vi "TallGuants_Main.vi"() -> ()   [LabVIEW 2017]
doc: "Use this template to build a simple state machine design pattern. Each state executes code and determines which state to transition to."
uses:
  controls/State.ctl
  controls/Data.ctl
  <vilib>/Utility/file.llb/Write Delimited Spreadsheet (string).vi
panel:
  in  "Sortir":bool caption="SALIR"
  out "Password":string
  out "EstatMaquina1":T1
  out "ParoEmergencia":bool caption="Paro de\nEmergencia"
  out "Retenida":bool
  out "Ensayo activo":bool caption="Prueba en marcha"
  out "Liberada":bool
  out "FCI":bool
  out "FCS":bool
  out "ADFet":bool
  out "CalibratgeDefor":dbl
  out "NProves":u8 caption="Longitud de corte"
  out "ValorSenseTara":dbl
  out "EntradesD":bool[](array[boolean])
  out "SortidesD":bool[](array[boolean])
  out "UI":bool[](array[boolean])
  in  "Vel.Maxima":sgl caption="Longitud de corte" format="%.1f"
  in  "Velocitat":sgl caption="Longitud de corte" format="%.1f"
  out "DadesAD":cluster{"Dades":sgl, "data":bool[]}
  in  "data":bool[](array[boolean])
  in  "Dades":sgl caption="Longitud de corte" format="%.1f"
  out "DigitalIn":refnum<vi>[](array[refnum])
  out "Tall":bool caption="Liberada"
  out "LongitudSenseTara":sgl caption="Longitud de corte" format="%.1f"
  out "Exit":bool
  out "FactorsUnitatsPendents_D":dbl[](array[numeric])
  out "ConversioUnitatsD":dbl[](array[numeric])=[1.0, 9.8756, 1000.0, 0.98]
  out "Tara":sgl caption="Longitud de corte" format="%.1f"
  in  "Table Control":string[][](table)
  in  "EnsayoNuevo":bool caption="Ensayo nuevo"
  in  "Calibracion":bool caption="Configuración"
  in  "Informe":bool
  in  "Fuerza de corte (N)":u16(ring) items=["1", "22", "33", "44", "5", "6", "7", "8", "9", "10", "11", "12", "13", "14", "15", "16", "17", "18", "19", "20", "21", "22", "23", "24", "25", "26", "27", "28", "29", "30"]
  in  "Down":bool
  in  "UP":bool caption="Up"
  in  "Cuchilla":bool
  in  "UnidadesD":u16(ring) caption="Unidades" items=["mm", "inch"]
  out "Longitud":sgl caption="Longitud de corte" format="%.2f"
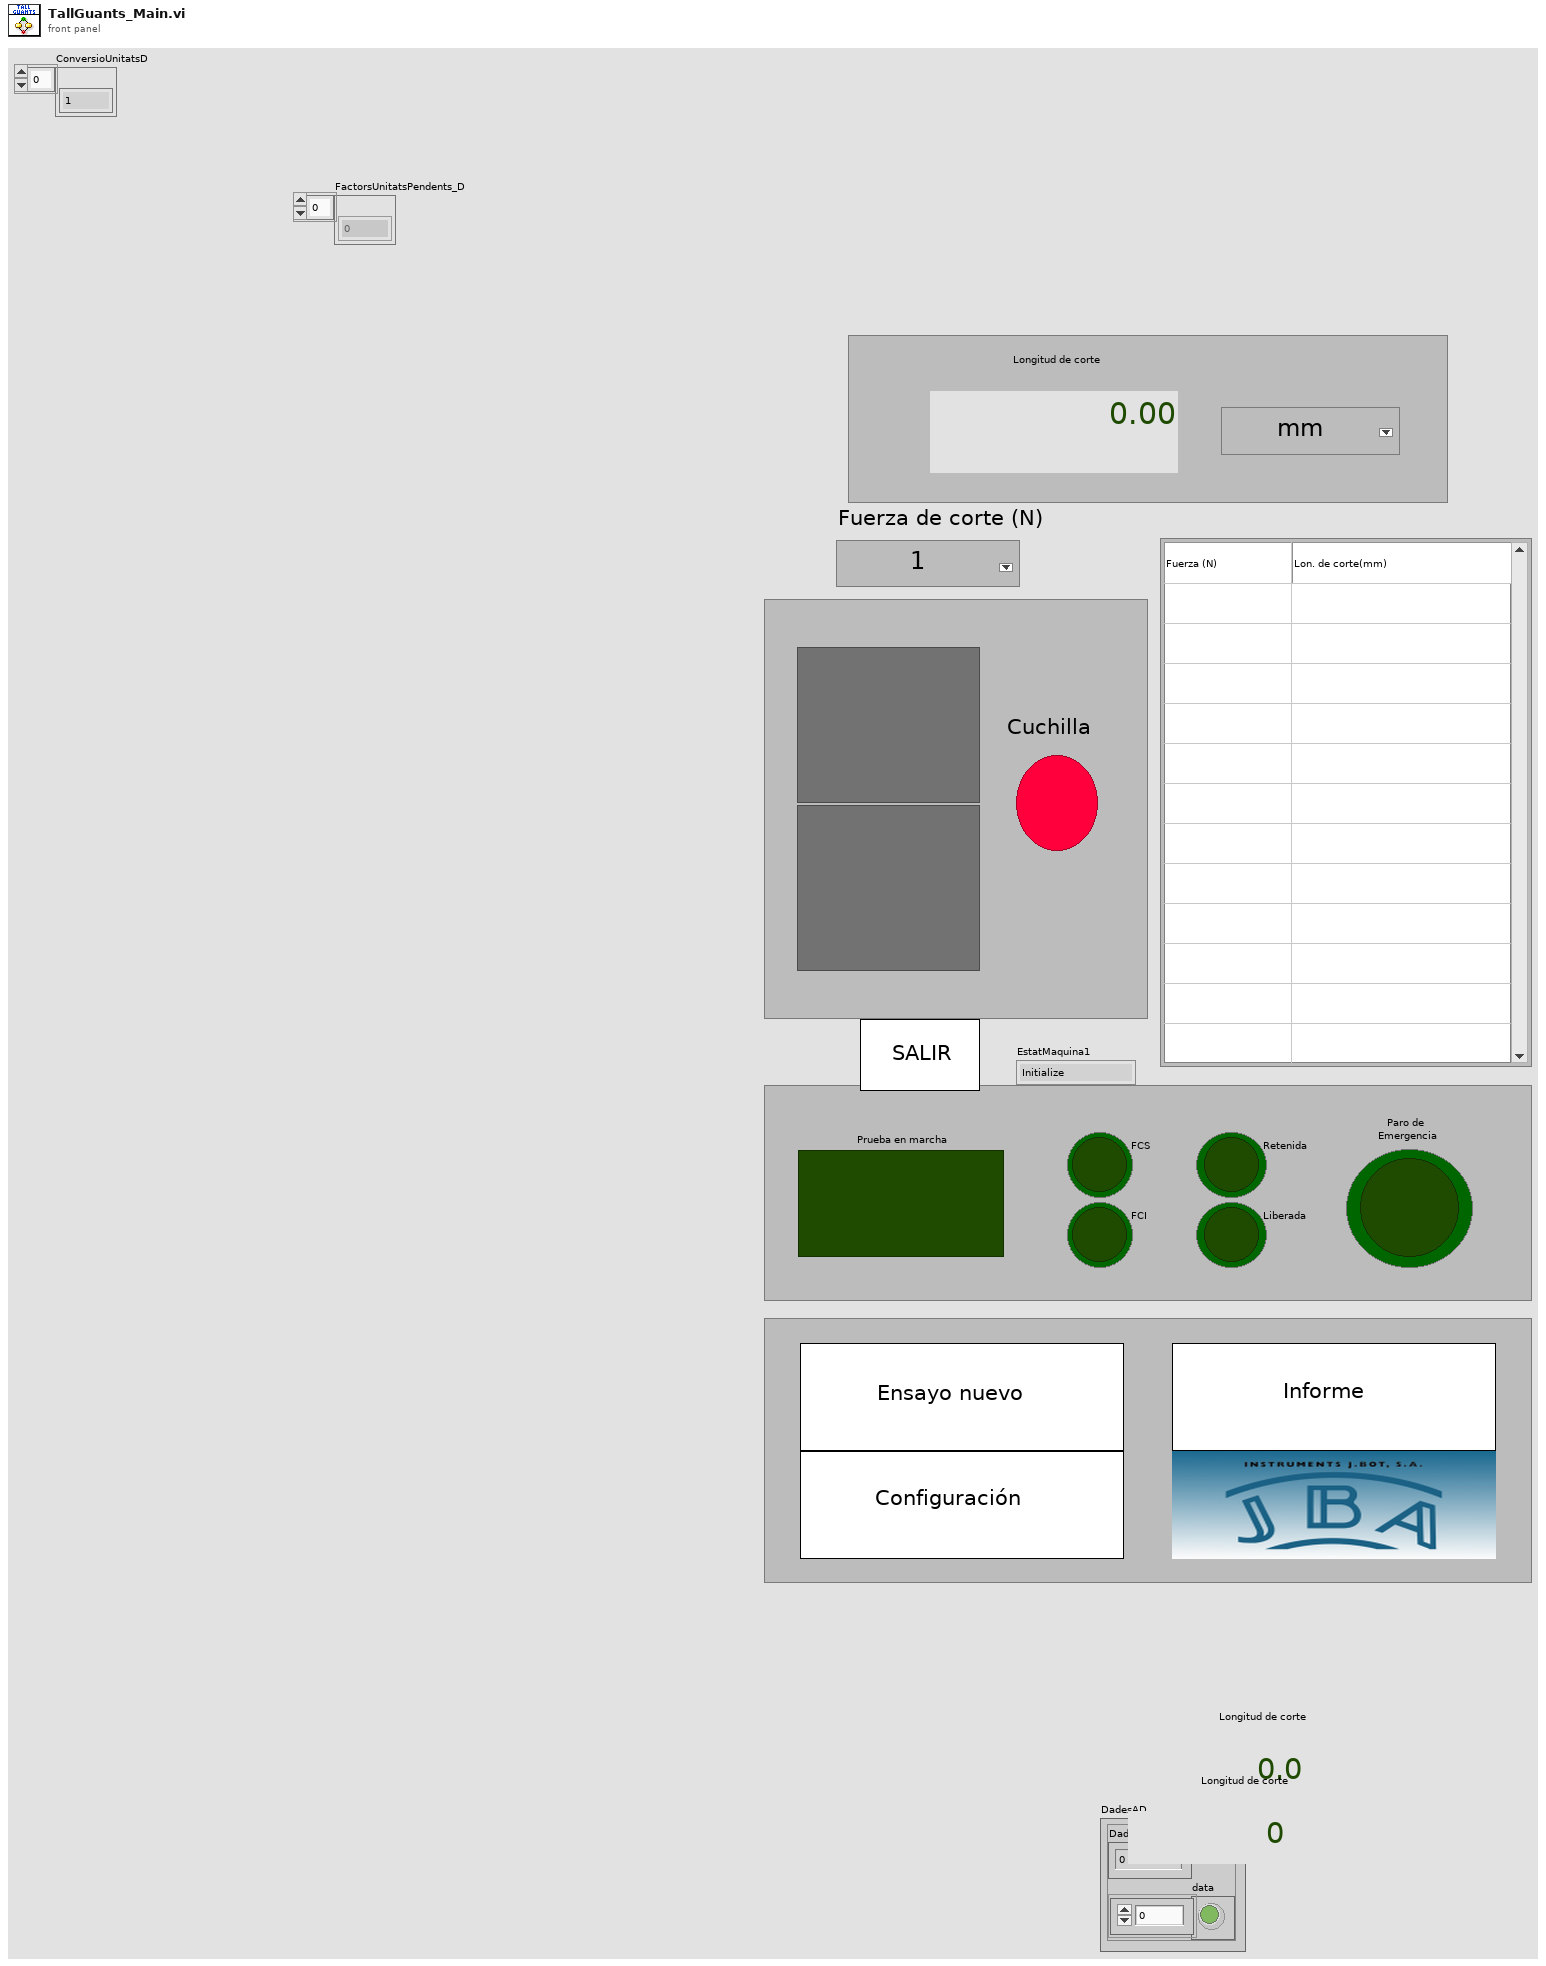
[diagram p1: front panel]
types:
  T1 = typedef "State.ctl" = enum16{"Initialize", "Wait for Event", "PreTest", "Test", "Puja", "Baixa", "Para", "Enclava_Ganiveta", "Des_Enclava_Ganiveta", "Tall_Fet", "AssaigNou", "Informe", "Calibració", "ParoEmergenciaActiu", "GanivetaDesenclavada", "Exit"}
  T2 = typedef "Data.ctl" = cluster{"Boolean <Replace Me>":bool, "String <Replace Me>":string, "EstatMaquina":T1}
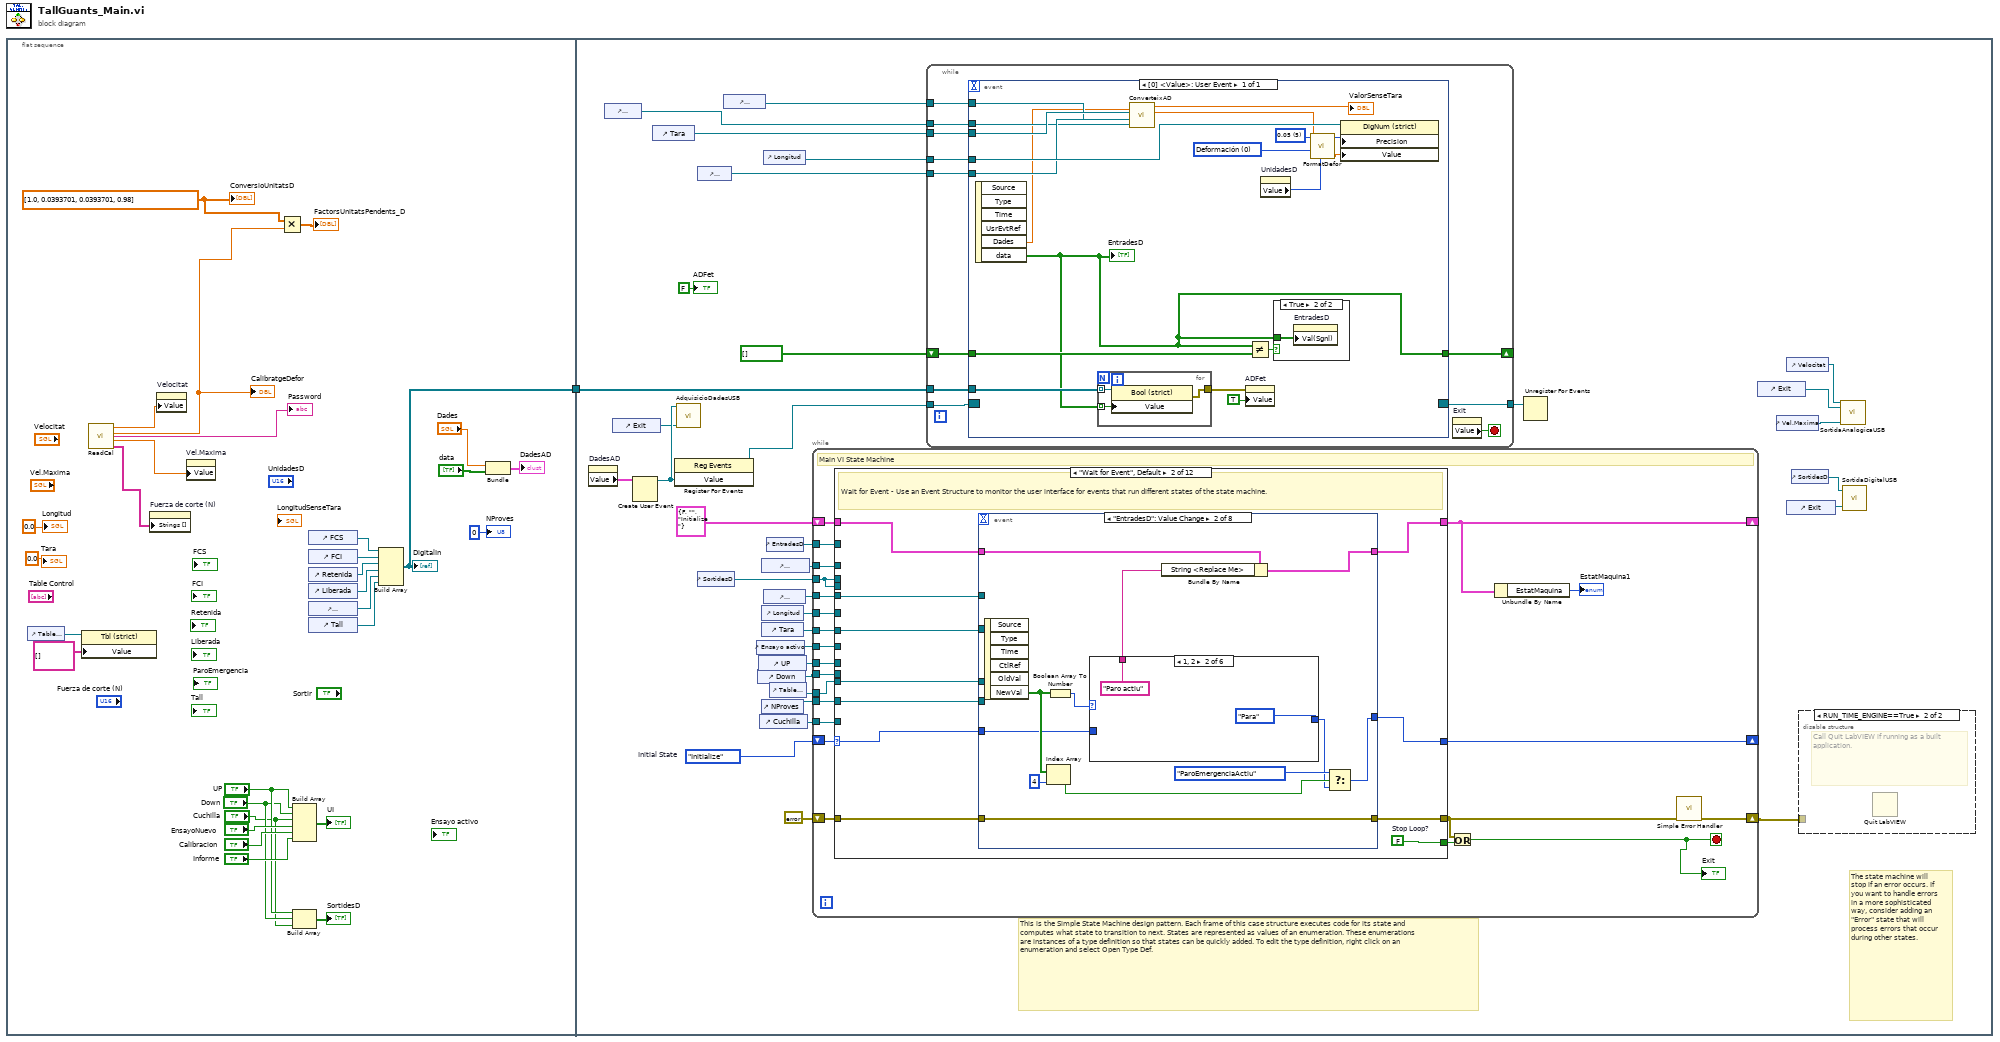
[diagram p0: block diagram]
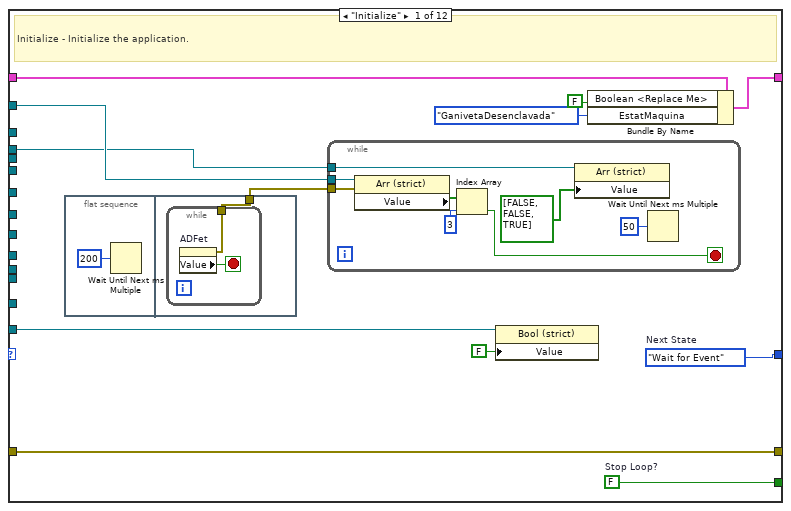
[diagram p4: hidden frame]
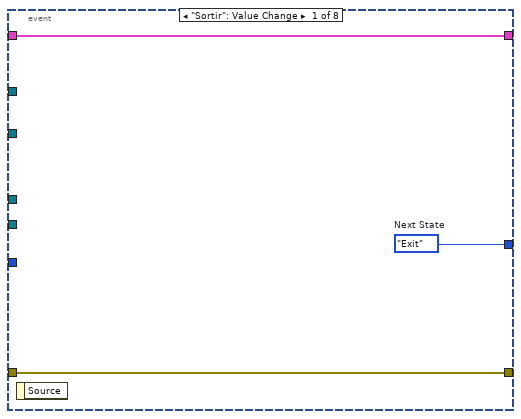
[diagram p5: hidden frame]
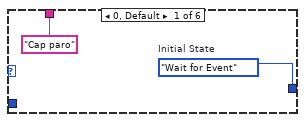
[diagram p6: hidden frame]
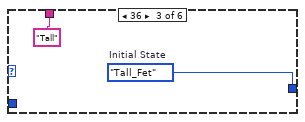
[diagram p7: hidden frame]
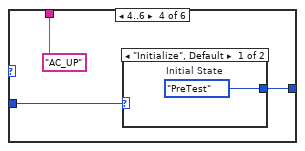
[diagram p8: hidden frame]
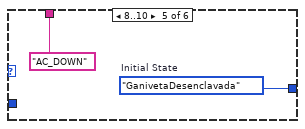
[diagram p10: hidden frame]
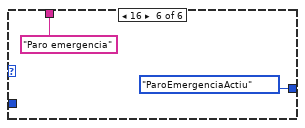
[diagram p11: hidden frame]
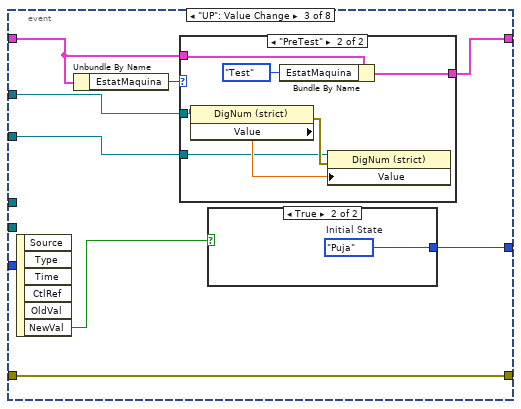
[diagram p12: hidden frame]
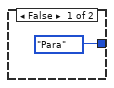
[diagram p14: hidden frame]
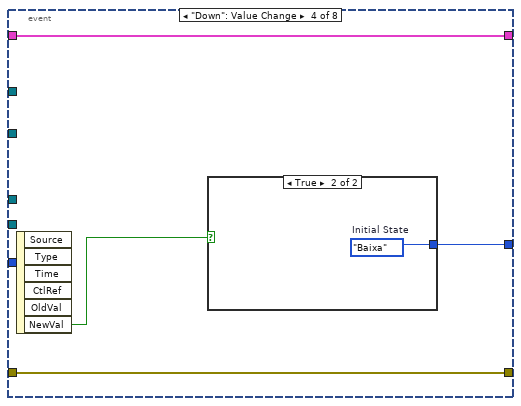
[diagram p15: hidden frame]
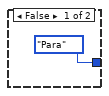
[diagram p16: hidden frame]
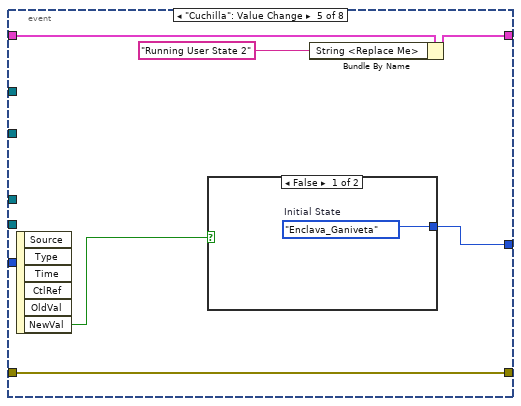
[diagram p17: hidden frame]
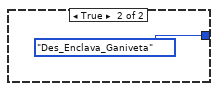
[diagram p18: hidden frame]
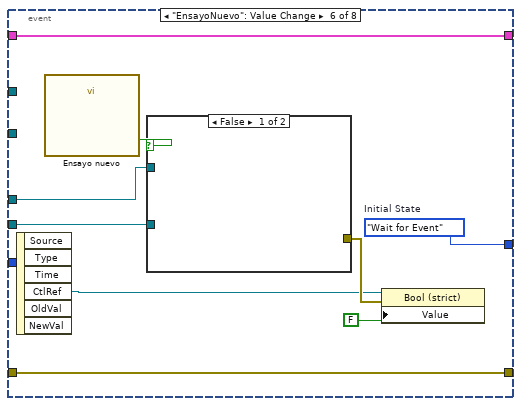
[diagram p19: hidden frame]
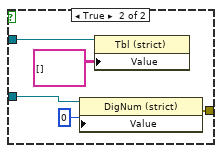
[diagram p20: hidden frame]
diagram:
  n1 = flat-sequence {
    tunnel: [w21] -> w1
    tunnel: w1 -> [w63]
    frame #0 {
      w28 = dbl[] [1.0, 0.0393701, 0.0393701, 0.98]
      n2 = control-ref of="Table Control"() -> (w4:refnum<vi>)
      n3 = property class="Tbl (strict)"(reference=w4, "Value"=string[][] []) -> ()  [unwired: 1 in, 2 out]
      n4 = call "ReadCal.vi"() -> ("Taula"=w5:string[], "VelocitatMaxima"=w7:dbl, "Deformacio"=w8:dbl, "Velocitat"=w6:dbl, "Password"=→"Password":string)  [unwired: 4 in]
      "CalibratgeDefor" <- w8
      n5 = property on="Fuerza de corte (N)" class="Ring (strict)"("Strings []"=w5) -> ()  [unwired: 2 in, 2 out]
      n6 = property on="Velocitat" class="DigNum (strict)"("Value"=w6) -> ()  [unwired: 2 in, 2 out]
      n7 = property on="Vel.Maxima" class="DigNum (strict)"("Value"=w7) -> ()  [unwired: 2 in, 2 out]
      n8 = Multiply(x=w28, y=w8) -> (x*y=→"FactorsUnitatsPendents_D":dbl[])
      n9 = Build Array("UP", "Down", "Cuchilla", "EnsayoNuevo", "Calibracion", "Informe") -> (→"UI":bool[])
      n10 = Build Array("UP", "Down", "Cuchilla") -> (→"SortidesD":bool[])
      n11 = control-ref of="FCS"() -> (w27:refnum<vi>)
      n12 = control-ref of="FCI"() -> (w26:refnum<vi>)
      n13 = control-ref of="Retenida"() -> (w25:refnum<vi>)
      n14 = control-ref of="Liberada"() -> (w24:refnum<vi>)
      n15 = control-ref of="ParoEmergencia"() -> (w23:refnum<vi>)
      n16 = control-ref of="Tall"() -> (w22:refnum<vi>)
      n17 = Build Array(w27, w26, w25, w24, w23, w22) -> (w21:refnum<vi>[])
      "DigitalIn" <- w21
      n18 = Bundle("Dades"="Dades", "data"="data") -> (→"DadesAD":cluster{"Dades":sgl, "data":bool[]})  [unwired: 1 in]
      "Longitud" <- sgl 0.0 ("Longitud")
      "Tara" <- sgl 0.0 ("Tara")
      "ConversioUnitatsD" <- w28
      "NProves" <- u8 0 ("NProves")
    }
    frame #1 {
      w53 = State."Initialize"  # Initial State
      # "The state machine will stop if an error occurs. If you want to handle errors in a more sophisticated way, consider adding an \"Error\" state that will process errors that occur during other states."
      # "This is the Simple State Machine design pattern. Each frame of this case structure executes code for its state and computes what state to transition to next. States are represented as values of an enumeration. These enumerations are instances of a type definition so that states can be quickly added. To edit the type definition, right click on an enumeration and select Open Type Def."
      n19 = property on="DadesAD" class="Clust (strict)"() -> ("Value"=w54:cluster{"Dades":sgl, "data":bool[]})  [unwired: 2 in, 2 out]
      n20 = control-ref of="FactorsUnitatsPendents_D"() -> (w59:refnum<vi>)
      n21 = control-ref of="Exit"() -> (w32:refnum<vi>)
      n22 = Create User Event(user event datatype=w54) -> (user event=w56:refnum<user-event>)  [unwired: 1 in, 1 out]
      n23 = control-ref of="Tara"() -> (w64:refnum<vi>)
      n24 = register-events(w56) -> (reference out=w55:refnum<event-registration>)  [unwired: 2 in, 1 out]
      n25 = call "AdquisicioDadesUSB.vi"("Stop"=w32, "user event out"=w56) -> ()  [unwired: 10 in]
      n26 = control-ref of="SortidesD"() -> (w47:refnum<vi>)
      n27 = control-ref of="UnidadesD"() -> (w58:refnum<vi>)
      n28 = control-ref of="LongitudSenseTara"() -> (w60:refnum<vi>)
      n29 = control-ref of="Ensayo activo"() -> (w43:refnum<vi>)
      n30 = control-ref of="Down"() -> (w38:refnum<vi>)
      n31 = control-ref of="UP"() -> (w39:refnum<vi>)
      n32 = control-ref of="Cuchilla"() -> (w37:refnum<vi>)
      n33 = control-ref of="ParoEmergencia"() -> (w35:refnum<vi>)
      n34 = control-ref of="NProves"() -> (w41:refnum<vi>)
      n35 = control-ref of="Longitud"() -> (w40:refnum<vi>)
      n36 = control-ref of="Tara"() -> (w45:refnum<vi>)
      n37 = control-ref of="Longitud"() -> (w65:refnum<vi>)
      n38 = control-ref of="ValorSenseTara"() -> (w44:refnum<vi>)
      n39 = control-ref of="EntradesD"() -> (w34:refnum<vi>)
      n40 = control-ref of="Table Control"() -> (w42:refnum<vi>)
      n41 = while {
        shift-right: [w106] -> _
        shift-left: T2 {"Boolean <Replace Me>"=FALSE, "String <Replace Me>"="", "EstatMaquina"=enum."Initialize"} ("Data") -> [w115]
        shift-right: [w102] -> w33
        shift-left: errorcluster {"status"=FALSE, "code"=0, "source"=""} ("error constant") -> [w121]
        shift-right: [w114] -> _
        shift-left: w53 -> [w118]
        tunnel: w47 -> [w100]
        tunnel: w45 -> [w117]
        tunnel: w44 -> [w116]
        tunnel: w43 -> [w113]
        tunnel: w42 -> [w112]
        tunnel: w41 -> [w111]
        tunnel: w40 -> [w110]
        tunnel: w39 -> [w109]
        tunnel: w38 -> [w108]
        tunnel: w37 -> [w107]
        tunnel: w35 -> [w104]
        tunnel: w34 -> [w103]
        stop <- w101 stop-if-true
        # "Main VI State Machine"
        n42 = case shown="\"Wait for Event\", Default" w118 {
          selector: w118 -> [_ w146 _ _ _ _ _ _ _ _ _ _]
          tunnel: [w133 w156 FALSE ("Stop Loop?") FALSE ("Stop Loop?") FALSE ("Stop Loop?") FALSE ("Stop Loop?") FALSE ("Stop Loop?") FALSE ("Stop Loop?") FALSE ("Stop Loop?") FALSE ("Stop Loop?") FALSE ("Stop Loop?") w375] -> w120
          tunnel: w115 -> [w132 w155 w266 w279 w287 w290 w304 w308 w329 w346 w366 w376]
          tunnel: [w131 w154 w266 w278 w286 w290 w304 w310 w327 w346 w365 w376] -> w106
          tunnel: w121 -> [w130 w153 w269 w281 w289 w296 w303 w313 w333 w345 w368 w374]
          tunnel: [w130 w152 w269 w281 w289 w296 w303 w313 w333 w345 w368 w374] -> w119
          tunnel: w100 -> [w124 _ w267 _ _ w294 w301 _ w326 _ _ _]
          tunnel: w117 -> [_ w149 _ _ _ _ _ _ _ _ _ _]
          tunnel: w116 -> [_ w150 _ _ _ _ _ _ _ _ _ _]
          tunnel: [w129 w151 w262 State."Para" ("(Value Not Used)") State."Wait for Event" ("(Value Not Used)") State."Wait for Event" ("Next State") w300 w311 w328 w343 w367 w373] -> w114
          tunnel: w113 -> [_ _ _ _ _ _ _ _ _ w342 w362 _]
          tunnel: w112 -> [_ w148 _ _ _ _ _ _ _ _ w357 _]
          tunnel: w111 -> [_ w147 _ _ _ _ _ _ _ _ w361 _]
          tunnel: w110 -> [_ _ _ _ _ _ _ _ _ _ w358 _]
          tunnel: w109 -> [_ _ _ _ _ _ _ w306 _ _ _ _]
          tunnel: w108 -> [_ _ _ _ _ _ _ w305 _ _ _ _]
          tunnel: w107 -> [w128 _ _ _ _ _ _ _ _ _ _ _]
          tunnel: w104 -> [_ _ _ _ _ w292 _ _ _ _ _ _]
          tunnel: w103 -> [w127 _ _ _ _ _ _ _ _ _ _ w371]
          tunnel: w100 -> [_ _ _ _ w282 _ _ w307 _ _ _ w372]
          frame "Initialize" {
            w133 = FALSE  # Stop Loop?
            w129 = State."Wait for Event"  # Next State
            # "Initialize - Initialize the application."
            n43 = flat-sequence {
              tunnel: [w135] -> w126
              frame #0 {
                n44 = Wait Until Next ms Multiple(millisecond multiple=u32 200) -> ()  [unwired: 1 out]
              }
              frame #1 {
                n45 = while {
                  tunnel: [w137] -> w135
                  stop <- w136 stop-if-true
                  n46 = property on="ADFet" class="Bool (strict)"() -> (error out=w137:errorcluster, "Value"=w136:bool)  [unwired: 2 in, 1 out]
                }
              }
            }
            n47 = while {
              tunnel: w127 -> [w145]
              tunnel: w126 -> [w144]
              tunnel: w124 -> [w140]
              stop <- w139 stop-if-true
              n48 = property class="Arr (strict)"(reference=w145, error in=w144) -> ("Value"=w142:bool[])  [unwired: 2 out]
              n49 = Index Array(array=w142, index=3) -> (element=w139:bool)
              n50 = property class="Arr (strict)"(reference=w140, "Value"=bool[] [FALSE, FALSE, TRUE] ("y")) -> ()  [unwired: 1 in, 2 out]
              n51 = Wait Until Next ms Multiple(millisecond multiple=u32 50) -> ()  [unwired: 1 out]
            }
            n52 = property class="Bool (strict)"(reference=w128, "Value"=FALSE) -> ()  [unwired: 1 in, 2 out]
            n53 = Bundle By Name(cluster=w132, "Boolean <Replace Me>"=FALSE ("Replace_Me_Boolean"), "EstatMaquina"=State."GanivetaDesenclavada") -> (w131:T2)
          }
          frame "Wait for Event", Default {
            w156 = FALSE  # Stop Loop?
            # "Wait for Event - Use an Event Structure to monitor the user interface for events that run different states of the state machine."
            n54 = event shown="[1] \"EntradesD\": Value Change" {
              selector: _ -> [_ _ _ _ _ _ _ _]
              dyn-events: _ -> [_ _ _ _ _ _ _ _]
              timeout: _ -> [_ _ _ _ _ _ _ _]
              tunnel: w155 -> [w159 w171 w190 w205 w216 w227 w242 w250]
              tunnel: [w159 w167 w189 w205 w215 w227 w242 w250] -> w154
              tunnel: w153 -> [w158 w170 w194 w208 w213 w226 w241 w249]
              tunnel: [w158 w170 w194 w208 w213 w226 w241 w249] -> w152
              tunnel: [w157 w162 w193 w207 w212 w222 w237 w248] -> w151
              tunnel: w150 -> [_ _ w188 _ _ _ _ _]
              tunnel: w149 -> [_ _ w187 _ _ _ _ _]
              tunnel: w148 -> [_ _ _ _ _ w224 w240 _]
              tunnel: w147 -> [_ _ _ _ _ w223 _ _]
              tunnel: w146 -> [_ w161 _ _ _ _ _ _]
              event "Sortir": Value Change {
                w157 = State."Exit"  # Next State
                n55 = event-data() -> ()  [unwired: 1 in, 1 out]
              }
              event "EntradesD": Value Change {
                n56 = event-data() -> ("NewVal"=w166:bool[])  [unwired: 1 in, 5 out]
                n57 = Index Array(array=w166, index=4) -> (element=w164:bool)
                n58 = Boolean Array To Number(Boolean array=w166) -> (number=w169:u32)
                n59 = case shown="1, 2" w169 {
                  tunnel: ["Cap paro" ("Running User State 1") "Paro actiu" ("Running User State 1") "Tall" ("Running User State 1") "AC_UP" ("Running User State 1") "AC_DOWN" ("Running User State 1") "Paro emergencia" ("Running User State 1")] -> w168
                  tunnel: [w172 State."Para" ("Initial State") w176 w178 w183 State."ParoEmergenciaActiu" ("Initial State")] -> w160
                  tunnel: w161 -> [_ _ _ w179 _ _]
                  frame 0, Default {
                    w172 = State."Wait for Event"  # Initial State
                  }
                  frame 1, 2 {
                  }
                  frame 36 {
                    w176 = State."Tall_Fet"  # Initial State
                  }
                  frame 4..6 {
                    n60 = case shown="\"Initialize\", Default" w179 {
                      selector: w179 -> [_ w182]
                      tunnel: [w181 w182] -> w178
                      frame "Initialize", Default {
                        w181 = State."PreTest"  # Initial State
                      }
                      frame "Test" {
                      }
                    }
                  }
                  frame 8..10 {
                    w183 = State."GanivetaDesenclavada"  # Initial State
                  }
                  frame 16 {
                  }
                }
                n61 = Bundle By Name(cluster=w171, "String <Replace Me>"=w168) -> (w167:T2)
                n62 = Select(t=State."ParoEmergenciaActiu" ("Initial State"), s=w164, f=w160) -> (s? t:f=w162:T1)
              }
              event "UP": Value Change {
                n63 = event-data() -> ("NewVal"=w192:bool)  [unwired: 1 in, 5 out]
                n64 = Unbundle By Name(w190) -> ("EstatMaquina"=w191:T1)
                n65 = case shown="\"PreTest\"" w191 {
                  tunnel: w190 -> [w195 w202]
                  tunnel: [w195 w200] -> w189
                  tunnel: w188 -> [_ w197]
                  tunnel: w187 -> [_ w196]
                  frame "Initialize", Default {
                  }
                  frame "PreTest" {
                    n66 = property class="DigNum (strict)"(reference=w197) -> (error out=w199:errorcluster, "Value"=w198:dbl)  [unwired: 1 in, 1 out]
                    n67 = Bundle By Name(cluster=w202, "EstatMaquina"=State."Test") -> (w200:T2)
                    n68 = property class="DigNum (strict)"(reference=w196, error in=w199, "Value"=w198) -> ()  [unwired: 2 out]
                  }
                }
                n69 = case shown="True" w192 {
                  tunnel: [State."Para" ("Initial State") w204] -> w193
                  frame False {
                  }
                  frame True {
                    w204 = State."Puja"  # Initial State
                  }
                }
              }
              event "Down": Value Change {
                n70 = event-data() -> ("NewVal"=w206:bool)  [unwired: 1 in, 5 out]
                n71 = case shown="True" w206 {
                  tunnel: [State."Para" ("Initial State") w210] -> w207
                  frame False {
                  }
                  frame True {
                    w210 = State."Baixa"  # Initial State
                  }
                }
              }
              event "Cuchilla": Value Change {
                n72 = event-data() -> ("NewVal"=w211:bool)  [unwired: 1 in, 5 out]
                n73 = case shown="False" w211 {
                  tunnel: [w217 State."Des_Enclava_Ganiveta" ("Initial State")] -> w212
                  frame False {
                    w217 = State."Enclava_Ganiveta"  # Initial State
                  }
                  frame True {
                  }
                }
                n74 = Bundle By Name(cluster=w216, "String <Replace Me>"="Running User State 2" ("Running User State 2")) -> (w215:T2)
              }
              event "EnsayoNuevo": Value Change {
                w222 = State."Wait for Event"  # Initial State
                n75 = event-data() -> ("CtlRef"=w219:refnum<vi>)  [unwired: 1 in, 5 out]
                n76 = call "Ensayo nuevo"() -> ("OK"=w225:bool)  [unwired: 18 in, 1 out]
                n77 = case shown="False" w225 {
                  tunnel: w224 -> [_ w232]
                  tunnel: w223 -> [_ w230]
                  tunnel: [_ w228] -> w221
                  frame False {
                  }
                  frame True {
                    n78 = property class="DigNum (strict)"(reference=w230, "Value"=u8 0) -> (error out=w228:errorcluster)  [unwired: 1 in, 1 out]
                    n79 = property class="Tbl (strict)"(reference=w232, "Value"=string[][] []) -> ()  [unwired: 1 in, 2 out]
                  }
                }
                n80 = property class="Bool (strict)"(reference=w219, error in=w221, "Value"=FALSE) -> ()  [unwired: 2 out]
              }
              event "Informe": Value Change {
                (unwired) 0 ("disabled index (col)")
                w237 = State."Wait for Event"  # Initial State
                n81 = event-data() -> ()  [unwired: 1 in, 6 out]
                n82 = property class="Tbl (strict)"(reference=w240) -> ("Value"=w233:string[][])  [unwired: 1 in, 2 out]
                n83 = call <vilib>:"Application Directory.vi"() -> ("Application Directory"=w238:path)
                n84 = Build Path(base path=w238, name or relative path="InformeTall.csv") -> (appended path=w236:path)
                n85 = call-poly <vilib>:"Write Delimited Spreadsheet.vi"("file path (dialog if empty)"=w236, "2D data"=w233, "append to file? (new file:F)"=FALSE ("transpose? (no:F)"), "delimiter (\\t)"=";" ("delimiter (\\t)")) -> ()  [unwired: 10 in, 2 out]
              }
              event "Calibracion": Value Change {
                w248 = State."Wait for Event"  # Initial State
                n86 = event-data() -> ("CtlRef"=w247:refnum<vi>)  [unwired: 1 in, 5 out]
                n87 = property on="Password" class="Str"() -> ("Value"=w243:string)  [unwired: 2 in, 2 out]
                n88 = call "Password.vi"() -> ("Password"=w245:string)  [unwired: 17 in, 2 out]
                n89 = Equal?(x=w243, y=w245) -> (x = y?=w244:bool)
                n90 = property class="Bool (strict)"(reference=w247, "Value"=FALSE) -> ()  [unwired: 1 in, 2 out]
                n91 = case shown="True" w244 {
                  frame False {
                  }
                  frame True {
                    n92 = call "Calibratge.vi"() -> ("FuerzasCorte"=w252:string[], "OK ?"=w255:bool, "DeformacioOut"=w253:dbl, "VelocitatMaximaOut"=w254:dbl, "VelocitatMotorOut"=w256:dbl, "Password 2"=w251:string)  [unwired: 1 in]
                    n93 = case shown="True" w255 {
                      tunnel: w256 -> [_ w261]
                      tunnel: w254 -> [_ w260]
                      tunnel: w253 -> [_ w259]
                      tunnel: w252 -> [_ w258]
                      tunnel: w251 -> [_ w257]
                      frame False {
                      }
                      frame True {
                        n94 = property on="Fuerza de corte (N)" class="Ring (strict)"("Strings []"=w258) -> ()  [unwired: 2 in, 2 out]
                        n95 = property on="Password" class="Str"("Value"=w257) -> ()  [unwired: 2 in, 2 out]
                        n96 = property on="Vel.Maxima" class="DigNum (strict)"("Value"=w260) -> ()  [unwired: 2 in, 2 out]
                        n97 = property on="CalibratgeDefor" class="DigNum (strict)"("Value"=w259) -> ()  [unwired: 2 in, 2 out]
                        n98 = property on="Velocitat" class="DigNum (strict)"("Value"=w261) -> ()  [unwired: 2 in, 2 out]
                      }
                    }
                  }
                }
              }
            }
          }
          frame "Puja" {
            n99 = Unbundle By Name(w266) -> ("EstatMaquina"=w265:T1)
            n100 = Equal?(x=w265, y=State."PreTest") -> (x = y?=w264:bool)
            n101 = case shown="False" w264 {
              tunnel: w267 -> [w270 w275]
              tunnel: [State."Wait for Event" ("Next State") State."Test" ("Next State")] -> w262
              frame False {
                n102 = property class="Arr (strict)"(reference=w270, "Value"=bool[] [TRUE, FALSE, FALSE] ("y")) -> ()  [unwired: 1 in, 2 out]
              }
              frame True {
                n103 = property class="Arr (strict)"(reference=w275, "Value"=bool[] [TRUE, FALSE, FALSE] ("y")) -> ()  [unwired: 1 in, 2 out]
              }
            }
          }
          frame "ParoEmergenciaActiu" {
            n104 = Bundle By Name(cluster=w279, "EstatMaquina"=State."ParoEmergenciaActiu") -> (w278:T2)
          }
          frame "GanivetaDesenclavada" {
            n105 = Bundle By Name(cluster=w287, "EstatMaquina"=State."GanivetaDesenclavada") -> (w286:T2)
            n106 = property class="Arr (strict)"(reference=w282, "Value"=bool[] [FALSE, FALSE, FALSE] ("y")) -> ()  [unwired: 1 in, 2 out]
          }
          frame "Baixa" {
            n107 = Unbundle By Name(w290) -> ("EstatMaquina"=w291:T1)
            n108 = case shown="\"PreTest\", \"Para\"" w291 {
              tunnel: w294 -> [_ w298]
              tunnel: w292 -> [_ _]
              frame "Initialize", Default {
              }
              frame "PreTest", "Para" {
                n109 = property class="Arr (strict)"(reference=w298, "Value"=bool[] [FALSE, TRUE, FALSE] ("y")) -> ()  [unwired: 1 in, 2 out]
              }
            }
          }
          frame "Enclava_Ganiveta", "Des_Enclava_Ganiveta" {
            w300 = State."Wait for Event"  # Initial State
            n110 = property class="Arr (strict)"(reference=w301, "Value"=bool[] [FALSE, FALSE, TRUE] ("y")) -> ()  [unwired: 1 in, 2 out]
          }
          frame "Para" {
            w311 = State."Wait for Event"  # Initial State
            n111 = Unbundle By Name(w308) -> ("EstatMaquina"=w309:T1)
            n112 = case shown="\"Initialize\", Default" w309 {
              tunnel: w308 -> [w321 w325]
              tunnel: [w322 w324] -> w310
              tunnel: w307 -> [w318 _]
              tunnel: w306 -> [w316 _]
              tunnel: w305 -> [w315 _]
              frame "Initialize", Default {
                w314 = FALSE ("Ensayo activo")
                w319 = FALSE ("Ensayo activo")
                n113 = property class="Bool (strict)"(reference=w316, "Value"=w314) -> ()  [unwired: 1 in, 2 out]
                n114 = property class="Bool (strict)"(reference=w315, "Value"=w314) -> ()  [unwired: 1 in, 2 out]
                n115 = property class="Arr (strict)"(reference=w318, "Value"=bool[] [FALSE, FALSE, FALSE]) -> ()  [unwired: 1 in, 2 out]
                n116 = property on="Ensayo activo" class="Bool (strict)"("Value"=w319) -> ()  [unwired: 2 in, 2 out]
                n117 = property on="UP" class="Bool (strict)"("Value"=w319) -> ()  [unwired: 2 in, 2 out]
                n118 = property on="Down" class="Bool (strict)"("Value"=w319) -> ()  [unwired: 2 in, 2 out]
                n119 = Bundle By Name(cluster=w321, "EstatMaquina"=State."Para") -> (w322:T2)
              }
              frame "Test" {
                n120 = Bundle By Name(cluster=w325, "EstatMaquina"=State."PreTest") -> (w324:T2)
              }
            }
          }
          frame "PreTest" {
            w328 = State."Wait for Event"  # Next State
            # "PreTest  -"
            n121 = Unbundle By Name(w329) -> ("String <Replace Me>"=w331:string)
            n122 = Equal?(x=w331, y="AC_UP") -> (x = y?=w332:bool)
            n123 = case shown="True" w332 {
              tunnel: w329 -> [w335 w340]
              tunnel: [w335 w338] -> w327
              tunnel: w326 -> [_ w336]
              frame False {
              }
              frame True {
                n124 = property class="Arr (strict)"(reference=w336, "Value"=bool[] [FALSE, FALSE, FALSE]) -> ()  [unwired: 1 in, 2 out]
                n125 = Bundle By Name(cluster=w340, "EstatMaquina"=State."PreTest") -> (w338:T2)
              }
            }
          }
          frame "Test" {
            w343 = State."Wait for Event"  # Next State
            n126 = property class="Bool (strict)"(reference=w342, "Value"=TRUE) -> ()  [unwired: 1 in, 2 out]
          }
          frame "Tall_Fet" {
            w364 = State."Tall_Fet"  # Next State
            w367 = State."Para"  # Next State
            # "User State 2 - Replace this state with functionality for your own application."
            n127 = property class="DigNum (strict)"(reference=w358) -> (error out=w356:errorcluster, "Value"=w355:sgl)  [unwired: 1 in, 1 out]
            n128 = property class="DigNum (strict)"(reference=w361) -> (reference out=w360:refnum<vi>, "Value"=w353:u8)  [unwired: 1 in, 1 out]
            n129 = property class="Bool (strict)"(reference=w362, "Value"=FALSE) -> ()  [unwired: 1 in, 2 out]
            n130 = property on="Fuerza de corte (N)" class="Ring (strict)"() -> ("RingText.Text"=w347:string)  [unwired: 2 in, 2 out]
            n131 = Bundle By Name(cluster=w366, "EstatMaquina"=w364) -> (w365:T2)
            n132 = Format Into String(format string="%4.2f", error in=w356, w355) -> (resulting string=w348:string)  [unwired: 1 in, 1 out]
            n133 = Increment(x=w353) -> (x+1=w359:u8)
            n134 = property class="Tbl (strict)"(reference=w357) -> (reference out=w350:refnum<vi>, "Value"=w352:string[][])  [unwired: 1 in, 1 out]
            n135 = property class="DigNum (strict)"(reference=w360, "Value"=w359) -> ()  [unwired: 1 in, 2 out]
            n136 = Build Array(w347, w348) -> (w351:string[])
            n137 = Insert Into Array(array=w352, new element=w351) -> (w349:string[][])  [unwired: 2 in]
            n138 = property class="Tbl (strict)"(reference=w350, "Value"=w349) -> ()  [unwired: 1 in, 2 out]
          }
          frame "Exit" {
            w375 = TRUE  # Stop Loop?
            w373 = State."Exit"  # (Value Not Used)
            # "Exit - Exit the application."
            n139 = flat-sequence {
              tunnel: w372 -> [w379]
              tunnel: w371 -> [w378]
              tunnel: [w377] -> w370
              tunnel: w370 -> [w389]
              frame #0 {
                n140 = while {
                  tunnel: w378 -> [w386]
                  tunnel: w379 -> [w382]
                  tunnel: [w380] -> w377
                  stop <- w381 stop-if-true
                  n141 = property class="Arr (strict)"(reference=w386) -> ("Value"=w384:bool[])  [unwired: 1 in, 2 out]
                  n142 = Index Array(array=w384, index=3) -> (element=w381:bool)
                  n143 = property class="Arr (strict)"(reference=w382, "Value"=bool[] [FALSE, FALSE, TRUE] ("y")) -> (reference out=w380:refnum<vi>)  [unwired: 1 in, 1 out]
                }
              }
              frame #1 {
                n144 = property class="Arr (strict)"(reference=w389, "Value"=bool[] [FALSE, FALSE, FALSE] ("y")) -> ()  [unwired: 1 in, 2 out]
                n145 = Wait Until Next ms Multiple(millisecond multiple=u32 50) -> ()  [unwired: 1 out]
              }
              frame #2 {
                n146 = Wait Until Next ms Multiple(millisecond multiple=u32 250) -> ()  [unwired: 1 out]
              }
            }
          }
        }
        n147 = Or(x=w119, y=w120) -> (x .or. y?=w101:bool)
        "Exit" <- w101
        n148 = Unbundle By Name(w106) -> ("EstatMaquina"=→"EstatMaquina1":T1)
        n149 = call <vilib>:"Simple Error Handler.vi"("error in (no error)"=w119) -> ("error out"=w102:errorcluster)  [unwired: 4 in, 4 out]
      }
      n150 = while {
        tunnel: w64 -> [w76]
        tunnel: w65 -> [w75]
        tunnel: w58 -> [w74]
        tunnel: w59 -> [w73]
        tunnel: w60 -> [w71]
        tunnel: w63 -> [w70]
        tunnel: [w68] -> w57
        tunnel: w55 -> [w69]
        shift-right: [w66] -> _
        shift-left: bool[] [] ("EntradesD") -> [w67]
        stop <- w72 stop-if-true
        n151 = event shown="[0] <Value>: User Event" {
          selector: w69 -> [_]
          dyn-events: [_] -> w68
          timeout: _ -> [_]
          tunnel: w76 -> [w95]
          tunnel: w75 -> [w94]
          tunnel: w74 -> [w93]
          tunnel: w73 -> [w92]
          tunnel: w71 -> [w91]
          tunnel: w70 -> [w82]
          tunnel: w67 -> [w81]
          tunnel: [w77] -> w66
          event User Event {
            w87 = i8 5 items=["0.1", "0.2", "0.5", "0.01", "0.02", "0.05", "0.001", "0.002", "0.005"] ("ResoExten")
            w88 = u16 0 items=["Deformación"] ("CaptadorD")
            n152 = event-data() -> ("Dades"=w84:sgl, "data"=w77:bool[])  [unwired: 1 in, 4 out]
            "EntradesD" <- w77
            n153 = for {
              tunnel: w82 -> [w99] mode=indexing
              tunnel: w77 -> [w98] mode=indexing
              tunnel: [w97] -> w78
              n154 = property class="Bool (strict)"(reference=w99, "Value"=w98) -> (error out=w97:errorcluster)  [unwired: 1 in, 1 out]
            }
            n155 = call "ConverteixAD.vi"("ValorSenseTara"=w91, "ValorAdquirid"=w84, "Unitats"=w93, "Tara"=w95, "FactorsUnitatsPendents"=w92) -> ("ValorActualAbs"=w90:dbl, "ValorSenseTara"=→"ValorSenseTara":dbl)  [unwired: 4 in, 1 out]
            n156 = property on="ADFet" class="Bool (strict)"(error in=w78, "Value"=TRUE ("ADFeta")) -> ()  [unwired: 1 in, 2 out]
            n157 = Not Equal?(x=w77, y=w81) -> (x != y?=w83:bool)
            n158 = property on="UnidadesD" class="Ring (strict)"() -> ("Value"=w86:u16)  [unwired: 2 in, 2 out]
            n159 = case shown="True" w83 {
              tunnel: w77 -> [_ w96]
              frame False {
              }
              frame True {
                n160 = property on="EntradesD" class="Arr (strict)"("Val(Sgnl)"=w96) -> ()  [unwired: 2 in, 2 out]
              }
            }
            n161 = call "FormatDefor.vi"("UnidadesD"=w86, "ValorIn"=w90, "CaptadorD"=w88, "ResoExten"=w87) -> ("ValorOut"=w89:dbl, "NDecimals"=w85:u8)  [unwired: 6 in]
            n162 = property class="DigNum (strict)"(reference=w94, "Precision"=w85, "Value"=w89) -> ()  [unwired: 1 in, 2 out]
          }
        }
        n163 = property on="Exit" class="Bool (strict)"() -> ("Value"=w72:bool)  [unwired: 2 in, 2 out]
      }
      n164 = Unregister For Events(event registration refnum=w57) -> ()  [unwired: 1 in, 1 out]
      n165 = control-ref of="Exit"() -> (w52:refnum<vi>)
      n166 = control-ref of="Vel.Maxima"() -> (w51:refnum<vi>)
      n167 = control-ref of="Velocitat"() -> (w50:refnum<vi>)
      n168 = control-ref of="Exit"() -> (w49:refnum<vi>)
      n169 = control-ref of="SortidesD"() -> (w46:refnum<vi>)
      n170 = disable-structure shown="RUN_TIME_ENGINE==True" {
        disable-tunnel: w33 -> [_ _]
        frame condition #0 (active) {
        }
        frame condition #1 {
          # "Call Quit LabVIEW if running as a built application."
          n171 = Quit LabVIEW() -> ()  [unwired: 1 in]
        }
      }
      n172 = call "SortidaAnalogicaUSB.vi"("VelocitatAssaig"=w50, "stop"=w52, "VelMaxima"=w51) -> ()  [unwired: 13 in]
      n173 = call "SortidaDigitalUSB.vi"("stop"=w49, "SortidesDigitals"=w46) -> ()  [unwired: 3 in]
      "ADFet" <- FALSE ("ADFeta")
    }
  }
